vi "Read inputs.vi"(9 "FlatSequence in":refnum<class "FlatSequence.lvclass">) -> (3 "FlatSequence out":refnum<class "FlatSequence.lvclass">, 4 "inputs":refnum<class "Terminal.lvclass">[](array[class]))   [LabVIEW 2014, in "FlatSequence.lvclass"]
uses:
  FlatSequence.lvclass
  Terminal/Terminal.lvclass
  FlatSequence.lvclass/FlatSequence.ctl
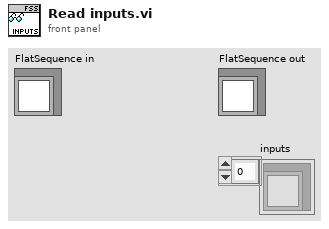
[diagram p1: front panel]
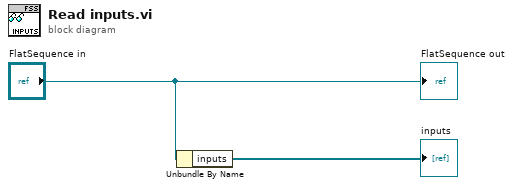
[diagram p0: block diagram]
diagram:
  n1 = Unbundle By Name("FlatSequence in") -> ("inputs"=→"inputs":refnum<class "Terminal.lvclass">[])
  "FlatSequence out" <- "FlatSequence in"
